vi "TestMessage.vi"(8 "error in":errorcluster, 10 "Payload (Guard Band)":string) -> (0 "error out":errorcluster, 2 "Output Bit Stream":i8[](array[numeric]))   [LabVIEW 2018]
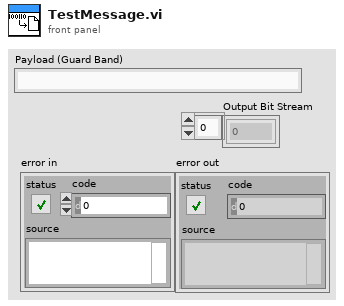
[diagram p1: front panel]
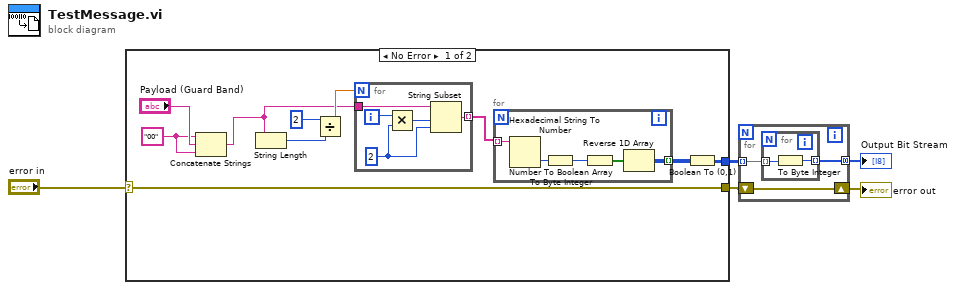
[diagram p0: block diagram]
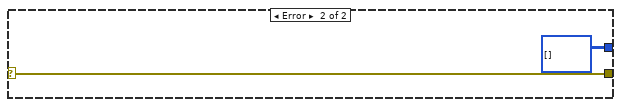
[diagram p2: hidden frame]
diagram:
  n1 = case shown="No Error" "error in" {
    selector: "error in" -> [w13 w26]
    tunnel: [w15 i16[][] []] -> w4
    tunnel: [w13 w26] -> w2
    frame No Error {
      w6 = "00" ("string")
      n2 = Concatenate Strings(w6, "Payload (Guard Band)", w6) -> (w7:string)
      n3 = String Length(string=w7) -> (length=w11:i32)
      n4 = Divide(x=w11, y=2) -> (x/y=w12:dbl)
      n5 = for {
        N: w12 -> [_]
        tunnel: w7 -> [w20]
        tunnel: [w19] -> w9 mode=indexing
        i -> [w18]
        w17 = 2 ("length (rest)")
        n6 = Multiply(x=w18, y=w17) -> (x*y=w16:i32)
        n7 = String Subset(string=w20, offset (0)=w16, length (rest)=w17) -> (substring=w19:string)
      }
      n8 = for {
        tunnel: w9 -> [w23] mode=indexing
        tunnel: [w21] -> w14 mode=indexing
        n9 = Hexadecimal String To Number(string=w23) -> (number=w24:u32)  [unwired: 2 in, 1 out]
        n10 = To Byte Integer(number=w24) -> (8bit integer=w22:i8)
        n11 = Number To Boolean Array(number=w22) -> (Boolean array=w25:bool[])
        n12 = Reverse 1D Array(array=w25) -> (reversed array=w21:bool[])
      }
      n13 = Boolean To (0,1)(Boolean=w14) -> (0, 1=w15:i16[][])
    }
    frame Error {
    }
  }
  n14 = for {
    tunnel: w4 -> [w30] mode=indexing
    tunnel: [w29] -> w3 mode=concatenating
    shift-right: [w28] -> w1
    shift-left: w2 -> [w28]
    n15 = for {
      tunnel: w30 -> [w32] mode=indexing
      tunnel: [w31] -> w29 mode=indexing
      n16 = To Byte Integer(number=w32) -> (8bit integer=w31:i8)
    }
  }
  "Output Bit Stream" <- w3
  "error out" <- w1
